vi "Add Widget to Container.vi"(5 "Container":refnum<class "QWidget.lvclass">, 8 "Error In":errorcluster, 9 "Label":string, 10 "Widget":refnum<class "QWidget.lvclass">, 11 "Abstract Widget Builder in":refnum<class "Abstract Widget Builder.lvclass">) -> (0 "Error Out":errorcluster, 3 "Abstract Widget Builder out":refnum<class "Abstract Widget Builder.lvclass">)   [LabVIEW 2014, in "Abstract Widget Builder.lvclass"]
doc: "Adds the specified Widget to the specified Container, using the specified Label.\n\nThis VI must be overridden by descendent classes.\n\n\nCopyright (c) 2019 Sze Howe Koh.\nThis code is licensed under the MIT license."
uses:
  Abstract Widget Builder.lvclass
  <vilib>/addons/LQ/Qt Widgets/QWidget/QWidget.lvclass
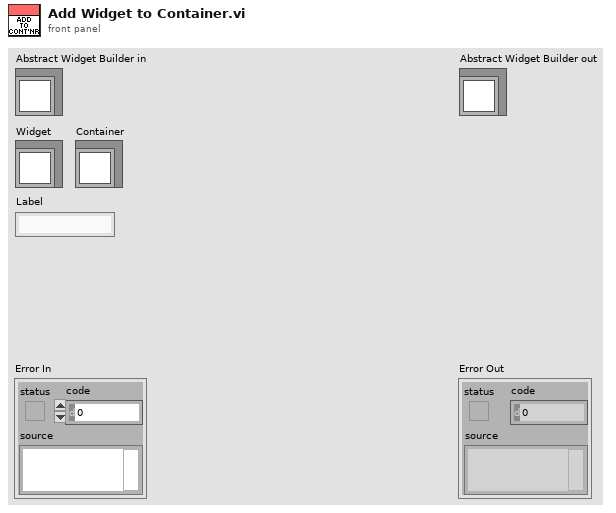
[diagram p1: front panel]
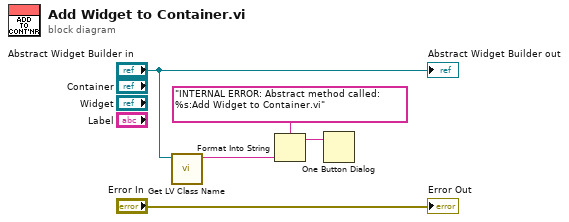
[diagram p0: block diagram]
diagram:
  n1 = call <vilib>:"Get LV Class Name.vi"("object"="Abstract Widget Builder in") -> ("class name"=w3:string)  [unwired: 9 in, 1 out]
  n2 = Format Into String(format string="INTERNAL ERROR: Abstract method called:  %s:Add Widget to Container.vi" ("message"), w3) -> (resulting string=w2:string)  [unwired: 2 in, 1 out]
  n3 = One Button Dialog(message=w2) -> ()  [unwired: 1 in, 1 out]
  "Error Out" <- "Error In"
  "Abstract Widget Builder out" <- "Abstract Widget Builder in"
